vi "_builtins_rect_next_column.vi"(10 "Indexes to Exclude":i32[](array[numeric]), 11 "Rects in":T1[](array[typedef])) -> (3 "Next Column Indexes":i32[](array[numeric]))   [LabVIEW 2019, in "Script.lvlib"]
doc: "Returns the next column of indexes using the top-left most rectangle as the reference object and filtering by rectangles to the left sorted from top-to-bottom.\n\nCreated by: Ryan Pacini"
uses:
  Script.lvlib
  <vilib>/Utility/miscctls.llb/LVRectTypeDef.ctl
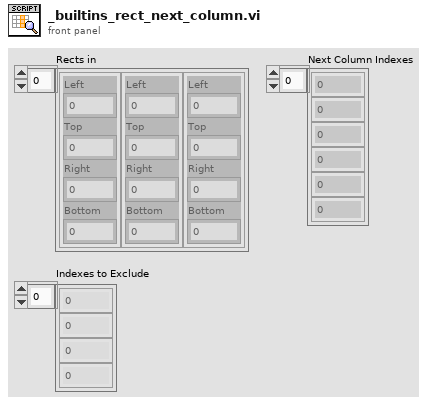
[diagram p1: front panel]
types:
  T1 = typedef "LVRectTypeDef.ctl" = cluster{"Left":i16, "Top":i16, "Right":i16, "Bottom":i16}
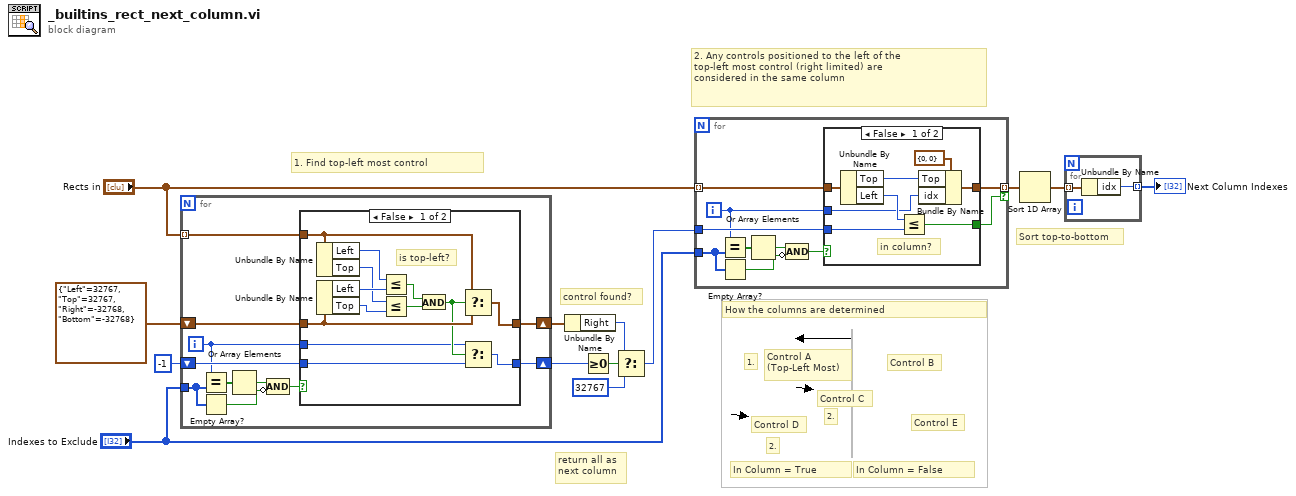
[diagram p0: block diagram]
diagram:
  # "return all as \nnext column"
  # "Sort top-to-bottom"
  # "2."
  # "2."
  # "1."
  # "In Column = False"
  # "In Column = True"
  # "How the columns are determined"
  # "Control E"
  # "Control B"
  # "Control D"
  # "Control C"
  # "Control A\n(Top-Left Most)"
  # "control found?"
  # "2. Any controls positioned to the left of the \ntop-left most control (right limited) are \nconsidered in the same column"
  # "1. Find top-left most control"
  n1 = for {
    tunnel: "Rects in" -> [w23] mode=indexing
    shift-right: [w24] -> w9
    shift-left: T1 {"Left"=32767, "Top"=32767, "Right"=-32768, "Bottom"=-32768} ("Rect") -> [w22]
    shift-right: [w21] -> w8
    shift-left: -1 -> [w20]
    tunnel: "Indexes to Exclude" -> [w15]
    i -> [w19]
    n2 = Equal?(x=w19, y=w15) -> (x = y?=w18:bool[])
    n3 = Empty Array?(array=w15) -> (empty?=w14:bool)
    n4 = Or Array Elements(Boolean array=w18) -> (logical OR=w17:bool)
    n5 = Compound Arithmetic op=AND(w17, invert w14) -> (w16:bool)
    n6 = case shown="False" w16 {
      tunnel: [w31 w39] -> w24
      tunnel: w23 -> [w30 _]
      tunnel: w22 -> [w29 w39]
      tunnel: w19 -> [w27 _]
      tunnel: [w26 w38] -> w21
      tunnel: w20 -> [w25 w38]
      frame False {
        # "is top-left?"
        n7 = Unbundle By Name(w30) -> ("Left"=w37:i16, "Top"=w34:i16)
        n8 = Unbundle By Name(w29) -> ("Left"=w36:i16, "Top"=w33:i16)
        n9 = Less Or Equal?(x=w37, y=w36) -> (x <= y?=w35:bool)
        n10 = Less Or Equal?(x=w34, y=w33) -> (x <= y?=w32:bool)
        n11 = And(x=w35, y=w32) -> (x .and. y?=w28:bool)
        n12 = Select(t=w30, s=w28, f=w29) -> (s? t:f=w31:T1)
        n13 = Select(t=w27, s=w28, f=w25) -> (s? t:f=w26:i32)
      }
      frame True {
        # "Exclude"
      }
    }
  }
  n14 = Unbundle By Name(w9) -> ("Right"=w6:i16)
  n15 = Greater Or Equal To 0?(x=w8) -> (x >= 0?=w7:bool)
  n16 = Select(t=w6, s=w7, f=i16 32767) -> (s? t:f=w5:i16)
  n17 = for {
    tunnel: "Rects in" -> [w49] mode=indexing
    tunnel: w5 -> [w48]
    tunnel: [w47] -> w13 mode=indexing if=w46
    tunnel: "Indexes to Exclude" -> [w41]
    i -> [w44]
    n18 = Equal?(x=w44, y=w41) -> (x = y?=w45:bool[])
    n19 = Empty Array?(array=w41) -> (empty?=w43:bool)
    n20 = Or Array Elements(Boolean array=w45) -> (logical OR=w42:bool)
    n21 = Compound Arithmetic op=AND(w42, invert w43) -> (w40:bool)
    n22 = case shown="False" w40 {
      tunnel: w49 -> [w57 _]
      tunnel: w48 -> [w55 _]
      tunnel: [w53 _] -> w47
      tunnel: [w51 _] -> w46
      tunnel: w44 -> [w50 _]
      frame False {
        # "in column?"
        n23 = Unbundle By Name(w57) -> ("Top"=w54:i16, "Left"=w56:i16)
        n24 = Less Or Equal?(x=w56, y=w55) -> (x <= y?=w51:bool)
        n25 = Bundle By Name(cluster=cluster{"Top":i16, "idx":i32} {"Top"=0, "idx"=0}, "Top"=w54, "idx"=w50) -> (w53:cluster{"Top":i16, "idx":i32})
      }
      frame True {
        # "Exclude"
      }
    }
  }
  n26 = Sort 1D Array(array=w13) -> (sorted array=w12:cluster{"Top":i16, "idx":i32}[])
  n27 = for {
    tunnel: w12 -> [w59] mode=indexing
    tunnel: [w58] -> w10 mode=indexing
    n28 = Unbundle By Name(w59) -> ("idx"=w58:i32)
  }
  "Next Column Indexes" <- w10
